vi "peg_leg_state_setpoints.vi"(11 "peg_leg_state":T1=enum."down") -> (3 "setpoint":dbl)   [LabVIEW 2011]
uses:
  peg_leg_state.ctl
panel:
  in  "Peg Leg States":dbl[](array[numeric])=[0.0, 90.0, 0.0]
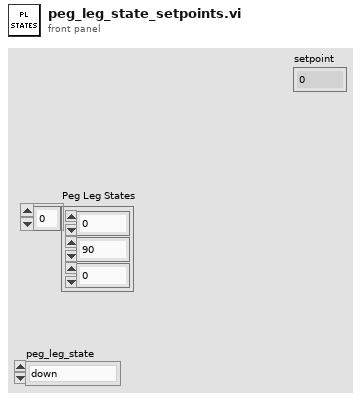
[diagram p1: front panel]
types:
  T1 = typedef "peg_leg_state.ctl" = enum16{"up", "down", "unfold", "manual"}
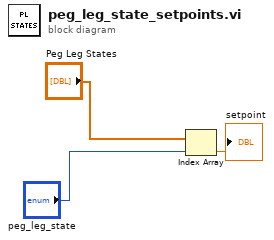
[diagram p0: block diagram]
diagram:
  n1 = Index Array(array="Peg Leg States", index="peg_leg_state") -> (element=→"setpoint":dbl)
